vi "DetPort3.vi"() -> ()   [LabVIEW 2013]
uses:
  SystemCode/SysControl/Slot.ctl
  <vilib>/Utility/error.llb/Error Cluster From Error Code.vi
  GlobalValue.vi
  <vilib>/ErrorRing/Error Ring.xnode
panel:
  out "检测结果":string
  in  "DET":bool
  out "Port":string[](array[string])
  in  "退出":bool
  out "error out":errorcluster caption="错误输出"
  in  "error in":errorcluster caption="错误输入（无错误）"
  # "1.插好连接线\n2.左侧和右侧测试工位放入并连接好T-BOX待测品。\n3.点击下面按钮等待检测通信接口完成。"
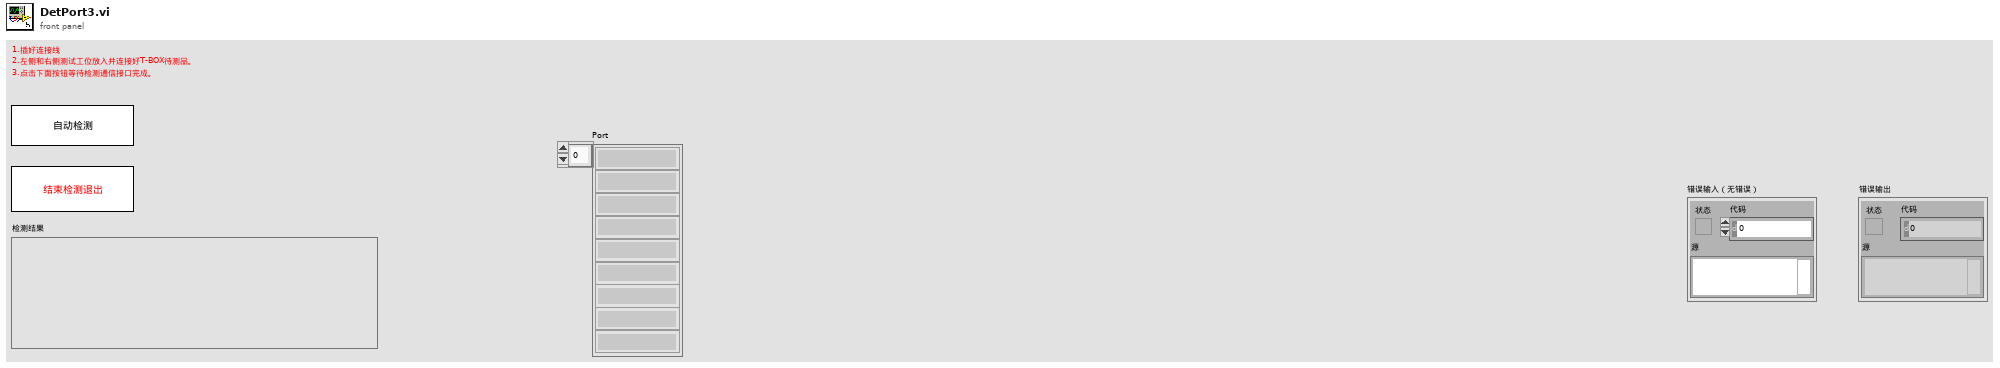
[diagram p1: front panel]
types:
  T1 = typedef "Slot.ctl" = enum16{"Slot1", "Slot2", "Slot3", "Slot4"}
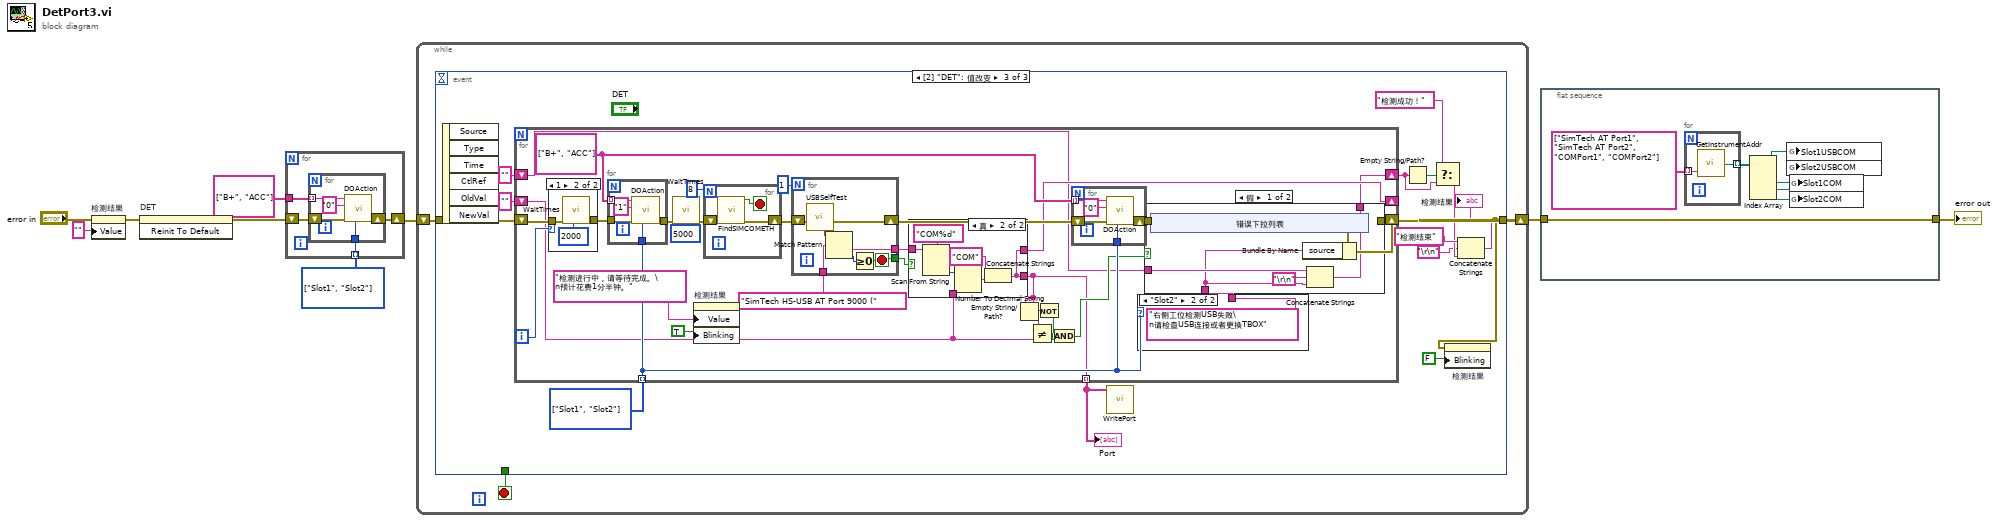
[diagram p0: block diagram]
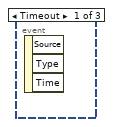
[diagram p2: hidden frame]
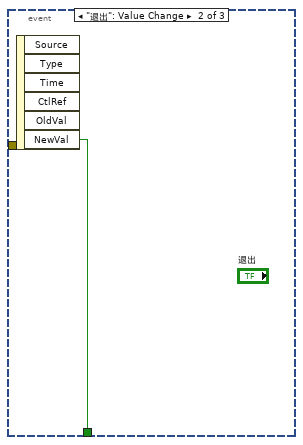
[diagram p3: hidden frame]
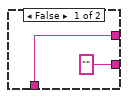
[diagram p4: hidden frame]
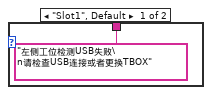
[diagram p6: hidden frame]
diagram:
  w7 = T1[] [enum."Slot1", enum."Slot2"] items=["Slot1", "Slot2", "Slot3", "Slot4"]
  n1 = property on="检测结果" class="Str"(error in="error in", "Value"="" ("检测结果")) -> (error out=w1:errorcluster)  [unwired: 1 in, 1 out]
  n2 = invoke on="DET" class="Bool" method="Reinit To Default"(error in=w1) -> (error out=w6:errorcluster)  [unwired: 2 in, 2 out]
  n3 = for {
    tunnel: string[] ["B+", "ACC"] -> [w13]
    tunnel: w7 -> [w12] mode=indexing
    shift-right: [w10] -> w5
    shift-left: w6 -> [w11]
    n4 = for {
      tunnel: w12 -> [w18]
      tunnel: w13 -> [w17] mode=indexing
      shift-right: [w14] -> w10
      shift-left: w11 -> [w15]
      n5 = call "DOAction.vi"("Slot"=w18, "error in"=w15, "State"="0", "CH"=w17) -> ("error out"=w14:errorcluster)  [unwired: 7 in]
    }
  }
  n6 = while {
    shift-right: [w19] -> w9
    shift-left: w5 -> [w20]
    stop <- w21 stop-if-true
    n7 = event shown="[2] \"DET\": 值改变" {
      selector: _ -> [_ _ _]
      dyn-events: _ -> [_ _ _]
      timeout: _ -> [_ _ _]
      tunnel: [_ w22 _] -> w21
      tunnel: w20 -> [_ _ w35]
      tunnel: [_ _ w24] -> w19
      event Timeout {
        n8 = event-data() -> ()  [unwired: 1 in, 3 out]
      }
      event "退出": Value Change {
        n9 = event-data() -> ("NewVal"=w22:bool)  [unwired: 1 in, 5 out]
      }
      event "DET": Value Change {
        w36 = T1[] [enum."Slot1", enum."Slot2"] items=["Slot1", "Slot2", "Slot3", "Slot4"]
        n10 = event-data() -> ()  [unwired: 1 in, 6 out]
        n11 = for {
          shift-right: [w57] -> w24
          shift-left: w35 -> [w55]
          tunnel: w36 -> [w61] mode=indexing
          tunnel: [w53] -> w34 mode=indexing
          shift-right: [w51] -> _
          shift-left: "" -> [w52]
          shift-right: [w49] -> w29
          shift-left: "" -> [w50]
          i -> [w56]
          w62 = string[] ["B+", "ACC"]
          n12 = case shown="1" w56 {
            tunnel: w55 -> [w84 w86]
            tunnel: [w84 w85] -> w54
            frame 0, Default {
            }
            frame 1 {
              n13 = call "WaitTimes.vi"("WaitTimes"=u32 2000, "error in (no error)"=w86) -> ("error out"=w85:errorcluster)  [unwired: 9 in]
            }
          }
          n14 = for {
            tunnel: w61 -> [w111]
            tunnel: w62 -> [w110] mode=indexing
            tunnel: w54 -> [w108]
            tunnel: [w107] -> w65
            n15 = call "DOAction.vi"("Slot"=w111, "error in"=w108, "State"="1", "CH"=w110) -> ("error out"=w107:errorcluster)  [unwired: 7 in]
          }
          n16 = call "WaitTimes.vi"("WaitTimes"=u32 5000, "error in (no error)"=w65) -> ("error out"=w41:errorcluster)  [unwired: 9 in]
          n17 = property on="检测结果" class="Str"("Value"="检测进行中，请等待完成。\n预计花费1分半钟。" ("检测结果"), "Blinking"=TRUE ("闪烁")) -> ()  [unwired: 2 in, 2 out]
          n18 = for {
            N: 8 -> [_]
            shift-right: [w67] -> w40
            shift-left: w41 -> [w68]
            stop <- w66 stop-if-true
            n19 = call "FindSIMCOMETH.vi"("error in (no error)"=w68) -> ("error out"=w67:errorcluster, "Result"=w66:bool)  [unwired: 9 in]
          }
          n20 = for {
            N: 1 -> [_]
            tunnel: [w81] -> w47
            tunnel: "SimTech HS-USB AT Port 9000 (" ("正则表达式") -> [w80]
            shift-right: [w79] -> w63
            shift-left: w40 -> [w83]
            tunnel: [w78] -> w45
            stop <- w78 stop-if-true
            n21 = call "USBSelfTest.vi"("error in (no error)"=w83) -> ("error out"=w79:errorcluster, "CmdOut"=w77:string)  [unwired: 8 in, 1 out]
            n22 = Match Pattern(string=w77, regular expression=w80) -> (after substring=w81:string, offset past match=w82:i32)  [unwired: 1 in, 2 out]
            n23 = Greater Or Equal To 0?(x=w82) -> (x >= 0?=w78:bool)
          }
          n24 = case shown="真" w45 {
            tunnel: w47 -> [_ w72]
            tunnel: ["" w71] -> w53
            tunnel: [w69 w71] -> w51
            tunnel: w52 -> [w69 _]
            frame False {
            }
            frame True {
              n25 = Scan From String(format string="COM%d" ("格式字符串"), input string=w72) -> (output 1=w75:i32)  [unwired: 3 in, 3 out]
              n26 = Number To Decimal String(number=w75) -> (decimal integer string=w73:string)  [unwired: 1 in]
              n27 = Concatenate Strings("COM" ("字符串"), w73) -> (w71:string)
            }
          }
          n28 = Empty String/Path?(string/path=w53) -> (empty?=w44:bool)
          n29 = Not Equal?(x=w53, y=w52) -> (x != y?=w42:bool)
          n30 = Not(x=w44) -> (.not. x?=w43:bool)
          n31 = And(x=w43, y=w42) -> (x .and. y?=w60:bool)
          n32 = for {
            tunnel: w61 -> [w106]
            tunnel: w62 -> [w105] mode=indexing
            shift-right: [w102] -> w58
            shift-left: w63 -> [w103]
            n33 = call "DOAction.vi"("Slot"=w106, "error in"=w103, "State"="0", "CH"=w105) -> ("error out"=w102:errorcluster)  [unwired: 7 in]
          }
          n34 = case shown="\"Slot2\"" w61 {
            tunnel: ["左侧工位检测USB失败\n请检查USB连接或者更换TBOX" ("消息") "右侧工位检测USB失败\n请检查USB连接或者更换TBOX" ("消息")] -> w59
            frame "Slot1", Default {
            }
            frame "Slot2" {
            }
          }
          n35 = case shown="假" w60 {
            tunnel: [w94 w101] -> w57
            tunnel: w58 -> [_ w101]
            tunnel: w59 -> [w91 _]
            tunnel: w50 -> [w93 w100]
            tunnel: [w92 w100] -> w49
            frame False {
              n36 = xnode "错误下拉列表"() -> ("错误输出"=w95:errorcluster)
              n37 = Bundle By Name(cluster=w95, "source"=w91) -> (w94:errorcluster)
              n38 = Concatenate Strings(w93, "\r\n", w91) -> (w92:string)
            }
            frame True {
            }
          }
        }
        "Port" <- w34
        n39 = call "WritePort.vi"("Port"=w34) -> ()  [unwired: 10 in, 1 out]
        n40 = Empty String/Path?(string/path=w29) -> (empty?=w32:bool)
        n41 = Select(t="检测成功！", s=w32, f=w29) -> (s? t:f=w27:string)
        n42 = property on="检测结果" class="Str"(error in=w24, "Blinking"=FALSE ("闪烁")) -> ()  [unwired: 1 in, 2 out]
        n43 = Concatenate Strings("检测结束" ("字符串"), "\r\n", w27) -> (→"检测结果":string)
      }
    }
  }
  n44 = flat-sequence {
    tunnel: w9 -> [w112]
    tunnel: [w112] -> w4
    frame #0 {
      n45 = for {
        tunnel: string[] ["SimTech AT Port1", "SimTech AT Port2", "COMPort1", "COMPort2"] -> [w120] mode=indexing
        tunnel: [w119] -> w114 mode=indexing
        n46 = call "GetInstrumentAddr.vi"("String"=w120) -> ("VISA session"=w119:refnum<visa-resource-name>)  [unwired: 1 out]
      }
      n47 = Index Array(array=w114) -> (element #1=w115:refnum<visa-resource-name>, element #2=w116:refnum<visa-resource-name>, element #3=w117:refnum<visa-resource-name>, element #4=w118:refnum<visa-resource-name>)  [unwired: 4 in]
      n48 = global write "GlobalValue.vi" "Slot1USBCOM"(w115) -> ()
      n49 = global write "GlobalValue.vi" "Slot2USBCOM"(w116) -> ()
      n50 = global write "GlobalValue.vi" "Slot1COM"(w117) -> ()
      n51 = global write "GlobalValue.vi" "Slot2COM"(w118) -> ()
    }
  }
  "error out" <- w4
